vi "ryerror_send.vi"(4 "clear error? (T)":bool=TRUE, 6 "error handler":refnum<queue>, 8 "error in (no error)":errorcluster) -> (0 "error out":errorcluster)   [LabVIEW 2017]
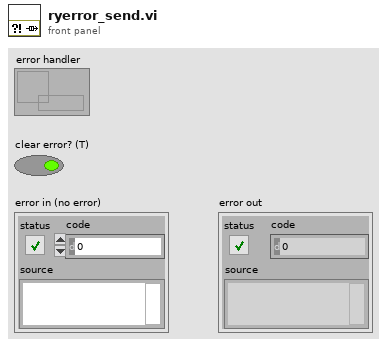
[diagram p1: front panel]
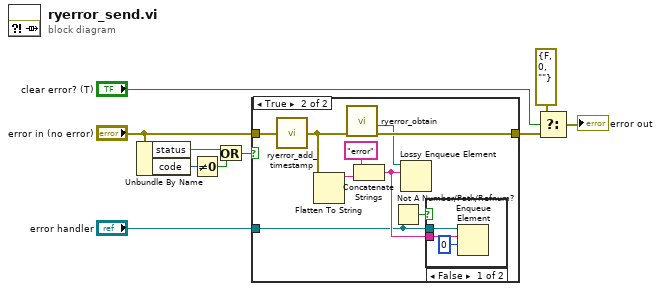
[diagram p0: block diagram]
diagram:
  n1 = Unbundle By Name("error in (no error)") -> ("status"=w9:bool, "code"=w8:i32)
  n2 = Not Equal To 0?(x=w8) -> (x != 0?=w7:bool)
  n3 = Or(x=w9, y=w7) -> (x .or. y?=w6:bool)
  n4 = case shown="True" w6 {
    tunnel: "error in (no error)" -> [w11 w12]
    tunnel: [w11 w19] -> w2
    tunnel: "error handler" -> [_ w14]
    frame False {
    }
    frame True {
      n5 = call "ryerror_add_timestamp.vi"("error in (no error)"=w12) -> ("error out"=w20:errorcluster)  [unwired: 8 in]
      n6 = Flatten To String(anything=w20) -> (data string=w17:string)  [unwired: 3 in, 2 out]
      n7 = call "ryerror_obtain.vi"("error in (no error)"=w20) -> ("error out"=w19:errorcluster, "error queue"=w18:refnum<queue>)  [unwired: 9 in]
      n8 = Concatenate Strings("error" ("string"), w17) -> (w15:string)
      n9 = Not A Number/Path/Refnum?(number/path/refnum=w14) -> (NaN/Path/Refnum?=w13:bool)
      n10 = Lossy Enqueue Element(queue=w18, element=w15) -> ()  [unwired: 1 in, 4 out]
      n11 = case shown="False" w13 {
        tunnel: w14 -> [w23 _]
        tunnel: w15 -> [w22 _]
        frame False {
          n12 = Enqueue Element(queue=w23, element=w22, timeout in ms (-1)=0) -> ()  [unwired: 1 in, 3 out]
        }
        frame True {
        }
      }
    }
  }
  n13 = Select(t=errorcluster {"status"=FALSE, "code"=0, "source"=""} ("error out"), s="clear error? (T)", f=w2) -> (s? t:f=→"error out":errorcluster)
